vi "Import Export - Load EC CD from XML.vi"(8 "Error In":errorcluster, 10 "Configuration File Path":path) -> (0 "Error Out":errorcluster, 3 "Temp File CD Out":T1 format="%.0x")   [LabVIEW 2017, in "Scan Engine Custom Device.lvlib"]
uses:
  Scan Engine Custom Device.lvlib
  <vilib>/NI Veristand/Custom Device API/Custom Device Item Ref.ctl
  <vilib>/NI/NI VeriStand Advanced SysDef API/_Types/SysDef.Export.ctl
  <vilib>/NI/NI VeriStand Advanced SysDef API/_Types/TreeItem.ctl
  <vilib>/NI/NI VeriStand Advanced SysDef API/_Types/TreeItem.Info.ctl
  <vilib>/NI Veristand/Custom Device API/Custom Device Channel.ctl
  <vilib>/NI Veristand/Custom Device API/Custom Device Channel Type.ctl
  <vilib>/NI Veristand/Custom Device API/Custom Device Waveform.ctl
  <vilib>/NI Veristand/Custom Device API/Custom Device Waveform DataType.ctl
  <vilib>/NI/NI VeriStand Advanced SysDef API/_Types/TreeItem.Property.ctl
  NationalInstruments.VeriStand.SystemDefinitionAPI
  Globals/Scan Engine GUIDs.vi
  NationalInstruments.VeriStand.SystemStorage
  <vilib>/NI/NI VeriStand Custom Device Import and Export Tool/ImportExport.lvlib
  <vilib>/NI/NI VeriStand Advanced SysDef API/SysDef API/Advanced System Definition.lvlib
  <vilib>/NI Veristand/Custom Device API/Custom Device API.lvlib
panel:
  in  "Temp File CD In":T1 format="%.0x"
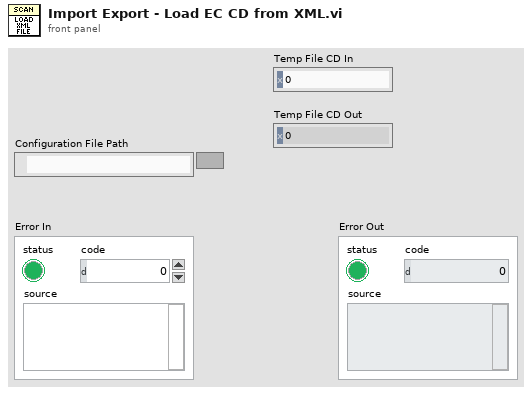
[diagram p1: front panel]
types:
  T1 = typedef "Custom Device API.lvlib/Custom Device Item Ref.ctl" = u64
  T2 = typedef "Advanced System Definition.lvlib/SysDef.Export.ctl" = cluster{"Version":string, "Tree":T3[]}
  T3 = typedef "Advanced System Definition.lvlib/TreeItem.ctl" = cluster{"Item Info":T4, "Parent Path":string[], "Properties":T9[]}
  T4 = typedef "Advanced System Definition.lvlib/TreeItem.Info.ctl" = cluster{"Name":string, "Description":string, "GUID":string, "Is Channel":bool, "Channel":T5, "Is Waveform":bool, "Waveform":T7}
  T5 = typedef "Custom Device API.lvlib/Custom Device Channel.ctl" = cluster{"Type":T6, "Units":string, "Default Value":dbl, "Faultable":bool, "Scalable":bool}
  T6 = typedef "Custom Device API.lvlib/Custom Device Channel Type.ctl" = enum16{"Input", "Output"}
  T7 = typedef "Custom Device API.lvlib/Custom Device Waveform.ctl" = cluster{"Data Type":T8, "Units":string}
  T8 = typedef "Custom Device API.lvlib/Custom Device Waveform DataType.ctl" = enum16{"Double", "Complex Double"}
  T9 = typedef "Advanced System Definition.lvlib/TreeItem.Property.ctl" = cluster{"Name":string, "Type":i32, "Value":variant}
  T10 = typedef "Custom Device API.lvlib/Custom Device Pointer.ctl" = refnum<k24>
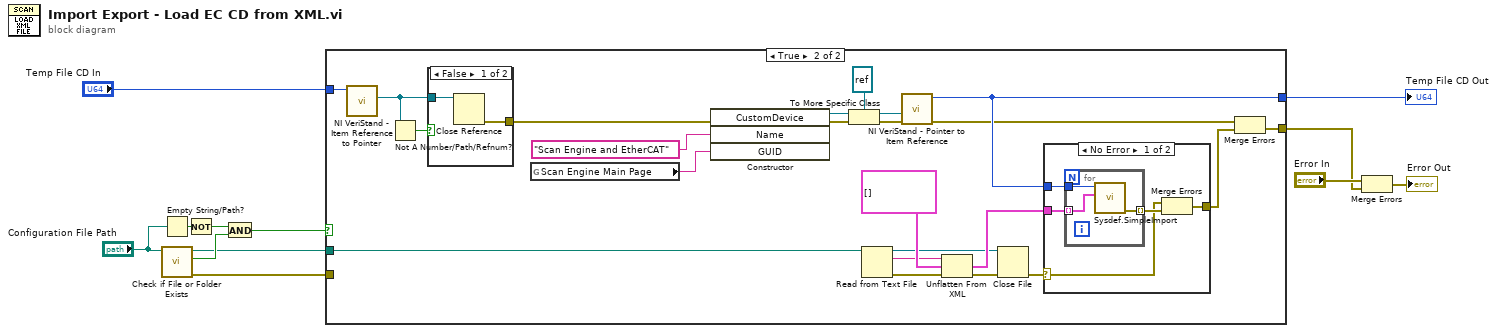
[diagram p0: block diagram]
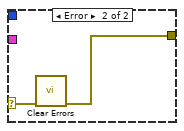
[diagram p4: hidden frame]
diagram:
  n1 = Empty String/Path?(string/path="Configuration File Path") -> (empty?=w8:bool)
  n2 = call <vilib>:"Check if File or Folder Exists.vi"("path"="Configuration File Path") -> ("error out"=w3:errorcluster, "file or folder exists?"=w7:bool, "dup path"=w5:path)  [unwired: 8 in]
  n3 = Not(x=w8) -> (.not. x?=w6:bool)
  n4 = And(x=w6, y=w7) -> (x .and. y?=w4:bool)
  n5 = case shown="True" w4 {
    tunnel: w5 -> [_ w33]
    tunnel: [w14 w29] -> w9
    tunnel: w3 -> [w14 _]
    tunnel: [w13 w16] -> w2
    tunnel: "Temp File CD In" -> [w13 w23]
    frame False {
    }
    frame True {
      n6 = call <vilib>:"NI VeriStand - Item Reference to Pointer.vi"("Item Ref in"=w23) -> ("Node Pointer"=w22:T10)  [unwired: 7 in, 3 out]
      n7 = Not A Number/Path/Refnum?(number/path/refnum=w22) -> (NaN/Path/Refnum?=w25:bool)
      n8 = case shown="False" w25 {
        tunnel: w22 -> [w39 _]
        tunnel: [w38 _] -> w24
        frame False {
          n9 = Close Reference(reference=w39) -> (error out=w38:errorcluster)  [unwired: 1 in]
        }
        frame True {
        }
      }
      n10 = global read "Scan Engine GUIDs.vi" "Scan Engine Main Page"() -> (w26:string)
      n11 = constructor class="CustomDevice"(error in=w24, "Name"="Scan Engine and EtherCAT", "GUID"=w26) -> (reference out=w18:refnum<k24>, error out=w17:errorcluster)  [unwired: 2 in, 3 out]
      n12 = To More Specific Class(target class=refnum<k24> refnum ("DeepCopy"), reference=w18, error in=w17) -> (specific class reference=w20:refnum<k24>, error out=w21:errorcluster)
      n13 = Read from Text File(file (use dialog)=w33) -> (refnum out=w32:refnum<file>, text=w34:string, error out=w35:errorcluster)  [unwired: 3 in, 1 out]
      n14 = call <vilib>:"NI VeriStand - Pointer to Item Reference.vi"("error in (no error)"=w21, "Node Pointer"=w20) -> ("error out"=w15:errorcluster, "Item Ref out"=w16:T1)  [unwired: 8 in]
      n15 = Unflatten From XML(xml string=w34, type=T2[] [], error in (no error)=w35) -> (value=w36:T2[], error out=w31:errorcluster)
      n16 = Close File(refnum=w32, error in=w31) -> (error out=w30:errorcluster)  [unwired: 1 out]
      n17 = case shown="No Error" w30 {
        selector: w30 -> [w40 w49]
        tunnel: w36 -> [w44 _]
        tunnel: w16 -> [w43 _]
        tunnel: [w41 w48] -> w28
        frame No Error {
          n18 = for {
            tunnel: w44 -> [w47] mode=indexing
            tunnel: w43 -> [w46]
            tunnel: [w45] -> w42 mode=indexing
            n19 = call <vilib>:"Sysdef.SimpleImport.vi"("SysDef"=w47, "NodeID"=w46) -> ("error out"=w45:errorcluster)  [unwired: 8 in, 1 out]
          }
          n20 = Merge Errors(w40, w42) -> (w41:errorcluster)
        }
        frame Error {
          n21 = call <vilib>:"Clear Errors.vi"("error in (no error)"=w49) -> ("error out"=w48:errorcluster)  [unwired: 5 in, 1 out]
        }
      }
      n22 = Merge Errors(w15, w28) -> (w29:errorcluster)
    }
  }
  "Temp File CD Out" <- w2
  n23 = Merge Errors("Error In", w9) -> (→"Error Out":errorcluster)
